vi "ExcelpathConvert.vi"(11 "输入字符串":string) -> (2 "路径":path, 3 "结果字符串":string)   [LabVIEW 2011]
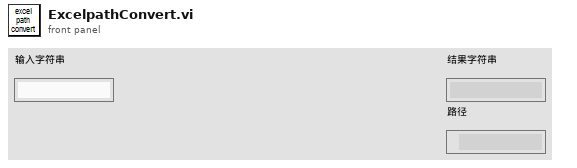
[diagram p1: front panel]
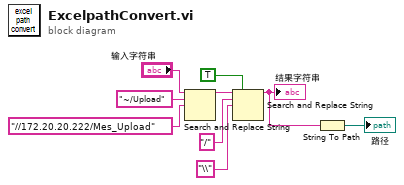
[diagram p0: block diagram]
diagram:
  n1 = Search and Replace String(input string="输入字符串", search string="~/Upload" ("搜索字符串"), replace string="//172.20.20.222/Mes_Upload" ("替换字符串(\"\")")) -> (result string=w7:string)  [unwired: 5 in, 3 out]
  n2 = Search and Replace String(replace all?=TRUE ("替换全部？(F)"), input string=w7, search string="/" ("搜索字符串"), replace string="\\" ("替换字符串(\"\")")) -> (result string=w2:string)  [unwired: 4 in, 3 out]
  "结果字符串" <- w2
  n3 = String To Path(string=w2) -> (path=→"路径":path)
